vi "UI_Set_ByZone_Stim._Control_State_on_Startup.vi"(8 "Error In":errorcluster, 9 "Regions to mark selected in":u8[](array[numeric]), 10 "All references cluster":T9, 11 "Settings cluster":T1={"Defaults"={"Default User"=0.0, "VISA Resource Name "=""}, "Recording and saving"={"Researcher name"="", "Name prefix"="", "Data post-processing"={"Filter type"=enum."Savitzky-Golay", "Length"=31, "Order"=3}, "Stop at"=0.0, "\"Stop at\" enabled"=FALSE, "Default save folder path"=path "", "Acquisition FPS"=enum."Max"}, "Geometry"={"Cage diameter, mm"=0, "Starting angle MIDFIELD"=0, "Starting angle BORDER"=0, "Radius, mm CENTER"=0, "Radius, mm MIDFIELD"=0, "N segments MIDFIELD"=0, "N segments BORDER"=0, "R-gap, mm"=0.0, "Bridge swap"=FALSE, "Bridge H. offset"=0.0, "Bridge V. offset"=0.0, "Twisted neck"=FALSE, "Alt. magn. orientation"=FALSE}, "IO parameters"={"IO general config."=0, "IO 1 configuration"=0, "IO 2 configuration"=0, "IO 3 configuration"=0, "IO 4 configuration"=0, "Activate ext. RS-232"=0, "IO inversion config."=0, "Sync capability"=1}, "Stimulus presets array"=[{"Event type"=0, "Dur., s"=0.0, "Stim., s"=0.0, "TTL out N"=1, "Set/Clear"=FALSE, "Stim. has been set"=FALSE}, {"Event type"=0, "Dur., s"=0.0, "Stim., s"=0.0, "TTL out N"=1, "Set/Clear"=FALSE, "Stim. has been set"=FALSE}, {"Event type"=0, "Dur., s"=0.0, "Stim., s"=0.0, "TTL out N"=1, "Set/Clear"=FALSE, "Stim. has been set"=FALSE}, {"Event type"=0, "Dur., s"=0.0, "Stim., s"=0.0, "TTL out N"=1, "Set/Clear"=FALSE, "Stim. has been set"=FALSE}, {"Event type"=0, "Dur., s"=0.0, "Stim., s"=0.0, "TTL out N"=1, "Set/Clear"=FALSE, "Stim. has been set"=FALSE}, {"Event type"=0, "Dur., s"=0.0, "Stim., s"=0.0, "TTL out N"=1, "Set/Clear"=FALSE, "Stim. has been set"=FALSE}, {"Event type"=0, "Dur., s"=0.0, "Stim., s"=0.0, "TTL out N"=1, "Set/Clear"=FALSE, "Stim. has been set"=FALSE}, {"Event type"=0, "Dur., s"=0.0, "Stim., s"=0.0, "TTL out N"=1, "Set/Clear"=FALSE, "Stim. has been set"=FALSE}, {"Event type"=0, "Dur., s"=0.0, "Stim., s"=0.0, "TTL out N"=1, "Set/Clear"=FALSE, "Stim. has been set"=FALSE}, {"Event type"=0, "Dur., s"=0.0, "Stim., s"=0.0, "TTL out N"=1, "Set/Clear"=FALSE, "Stim. has been set"=FALSE}, {"Event type"=0, "Dur., s"=0.0, "Stim., s"=0.0, "TTL out N"=1, "Set/Clear"=FALSE, "Stim. has been set"=FALSE}, {"Event type"=0, "Dur., s"=0.0, "Stim., s"=0.0, "TTL out N"=1, "Set/Clear"=FALSE, "Stim. has been set"=FALSE}, {"Event type"=0, "Dur., s"=0.0, "Stim., s"=0.0, "TTL out N"=1, "Set/Clear"=FALSE, "Stim. has been set"=FALSE}, {"Event type"=0, "Dur., s"=0.0, "Stim., s"=0.0, "TTL out N"=1, "Set/Clear"=FALSE, "Stim. has been set"=FALSE}], "Calibration parameters"={"Timing calibration sw/hw"=1.0, "True FPS"=80.0, "Disp. calibration info"=[]}, "Settings loaded OK"=FALSE} {"Calibration parameters"."Disp. calibration info"."Speed, µl per ms" format="%.3g"; "Calibration parameters"."True FPS" format="%.10g"; "Calibration parameters"."Timing calibration sw/hw" format="%.10g"; "Stimulus presets array"."Event type" items=["Stay for N seconds"]; "Stimulus presets array"."TTL out N" items=["1"=1, "2"=2, "1+2"=3]; "Recording and saving"."Data post-processing"."Order" min=3 max=11 step=2; "Recording and saving"."Data post-processing"."Length" min=5 max=301 step=2; "Geometry"."Cage diameter, mm" scale=0.0..340.0}) -> (0 "Error Out":errorcluster, 1 "Regions to mark selected out":u8[](array[numeric]), 2 "All references cluster out":T9, 3 "Regions set for tracking":u8[](array[numeric]), 5 "Settings cluster out":T1={"Defaults"={"Default User"=0.0, "VISA Resource Name "=""}, "Recording and saving"={"Researcher name"="", "Name prefix"="", "Data post-processing"={"Filter type"=enum."Savitzky-Golay", "Length"=31, "Order"=3}, "Stop at"=0.0, "\"Stop at\" enabled"=FALSE, "Default save folder path"=path "", "Acquisition FPS"=enum."Max"}, "Geometry"={"Cage diameter, mm"=0, "Starting angle MIDFIELD"=0, "Starting angle BORDER"=0, "Radius, mm CENTER"=0, "Radius, mm MIDFIELD"=0, "N segments MIDFIELD"=0, "N segments BORDER"=0, "R-gap, mm"=0.0, "Bridge swap"=FALSE, "Bridge H. offset"=0.0, "Bridge V. offset"=0.0, "Twisted neck"=FALSE, "Alt. magn. orientation"=FALSE}, "IO parameters"={"IO general config."=0, "IO 1 configuration"=0, "IO 2 configuration"=0, "IO 3 configuration"=0, "IO 4 configuration"=0, "Activate ext. RS-232"=0, "IO inversion config."=0, "Sync capability"=1}, "Stimulus presets array"=[{"Event type"=0, "Dur., s"=0.0, "Stim., s"=0.0, "TTL out N"=1, "Set/Clear"=FALSE, "Stim. has been set"=FALSE}, {"Event type"=0, "Dur., s"=0.0, "Stim., s"=0.0, "TTL out N"=1, "Set/Clear"=FALSE, "Stim. has been set"=FALSE}, {"Event type"=0, "Dur., s"=0.0, "Stim., s"=0.0, "TTL out N"=1, "Set/Clear"=FALSE, "Stim. has been set"=FALSE}, {"Event type"=0, "Dur., s"=0.0, "Stim., s"=0.0, "TTL out N"=1, "Set/Clear"=FALSE, "Stim. has been set"=FALSE}, {"Event type"=0, "Dur., s"=0.0, "Stim., s"=0.0, "TTL out N"=1, "Set/Clear"=FALSE, "Stim. has been set"=FALSE}, {"Event type"=0, "Dur., s"=0.0, "Stim., s"=0.0, "TTL out N"=1, "Set/Clear"=FALSE, "Stim. has been set"=FALSE}, {"Event type"=0, "Dur., s"=0.0, "Stim., s"=0.0, "TTL out N"=1, "Set/Clear"=FALSE, "Stim. has been set"=FALSE}, {"Event type"=0, "Dur., s"=0.0, "Stim., s"=0.0, "TTL out N"=1, "Set/Clear"=FALSE, "Stim. has been set"=FALSE}, {"Event type"=0, "Dur., s"=0.0, "Stim., s"=0.0, "TTL out N"=1, "Set/Clear"=FALSE, "Stim. has been set"=FALSE}, {"Event type"=0, "Dur., s"=0.0, "Stim., s"=0.0, "TTL out N"=1, "Set/Clear"=FALSE, "Stim. has been set"=FALSE}, {"Event type"=0, "Dur., s"=0.0, "Stim., s"=0.0, "TTL out N"=1, "Set/Clear"=FALSE, "Stim. has been set"=FALSE}, {"Event type"=0, "Dur., s"=0.0, "Stim., s"=0.0, "TTL out N"=1, "Set/Clear"=FALSE, "Stim. has been set"=FALSE}, {"Event type"=0, "Dur., s"=0.0, "Stim., s"=0.0, "TTL out N"=1, "Set/Clear"=FALSE, "Stim. has been set"=FALSE}, {"Event type"=0, "Dur., s"=0.0, "Stim., s"=0.0, "TTL out N"=1, "Set/Clear"=FALSE, "Stim. has been set"=FALSE}], "Calibration parameters"={"Timing calibration sw/hw"=1.0, "True FPS"=80.0, "Disp. calibration info"=[]}, "Settings loaded OK"=FALSE} {"Calibration parameters"."Disp. calibration info"."Speed, µl per ms" format="%.3g"; "Calibration parameters"."True FPS" format="%.10g"; "Calibration parameters"."Timing calibration sw/hw" format="%.10g"; "Stimulus presets array"."Event type" items=["Stay for N seconds"]; "Stimulus presets array"."TTL out N" items=["1"=1, "2"=2, "1+2"=3]; "Recording and saving"."Data post-processing"."Order" min=3 max=11 step=2; "Recording and saving"."Data post-processing"."Length" min=5 max=301 step=2; "Geometry"."Cage diameter, mm" scale=0.0..340.0})   [LabVIEW 2018, in "Tracker.lvlib"]
uses:
  Tracker.lvlib
  Controls/CTL_Settings_cluster.ctl
  Controls/CTL_Filter_selector.ctl
  Controls/CTL_Acquisition_speed_selector.ctl
  Controls/CTL_Segmented_plot_parameters.ctl
  Controls/CTL_IO_params_cluster.ctl
  Controls/CTL_Single_stimulus_setting.ctl
  Controls/CTL_Calibration_parameters.ctl
  Controls/CTL_Dispenser_calibration_info.ctl
  Controls/CTL_All_References.ctl
  Controls/CTL_Controls_References.ctl
  Controls/CTL_Indicators_References.ctl
  Controls/CTL_Panes_and_VIs_References.ctl
  Controls/CTL_Zones_control_and_indicator.ctl
panel:
  in  "Colors for Stim. setup":T13(array[cluster])=[{"Not Selected"=1143775, "Not Selected"=1143775}, {"Not Selected"=14517504, "Not Selected"=14517504}, {"Not Selected"=1976113, "Not Selected"=1976113}, {"Not Selected"=2575993, "Not Selected"=2575993}]
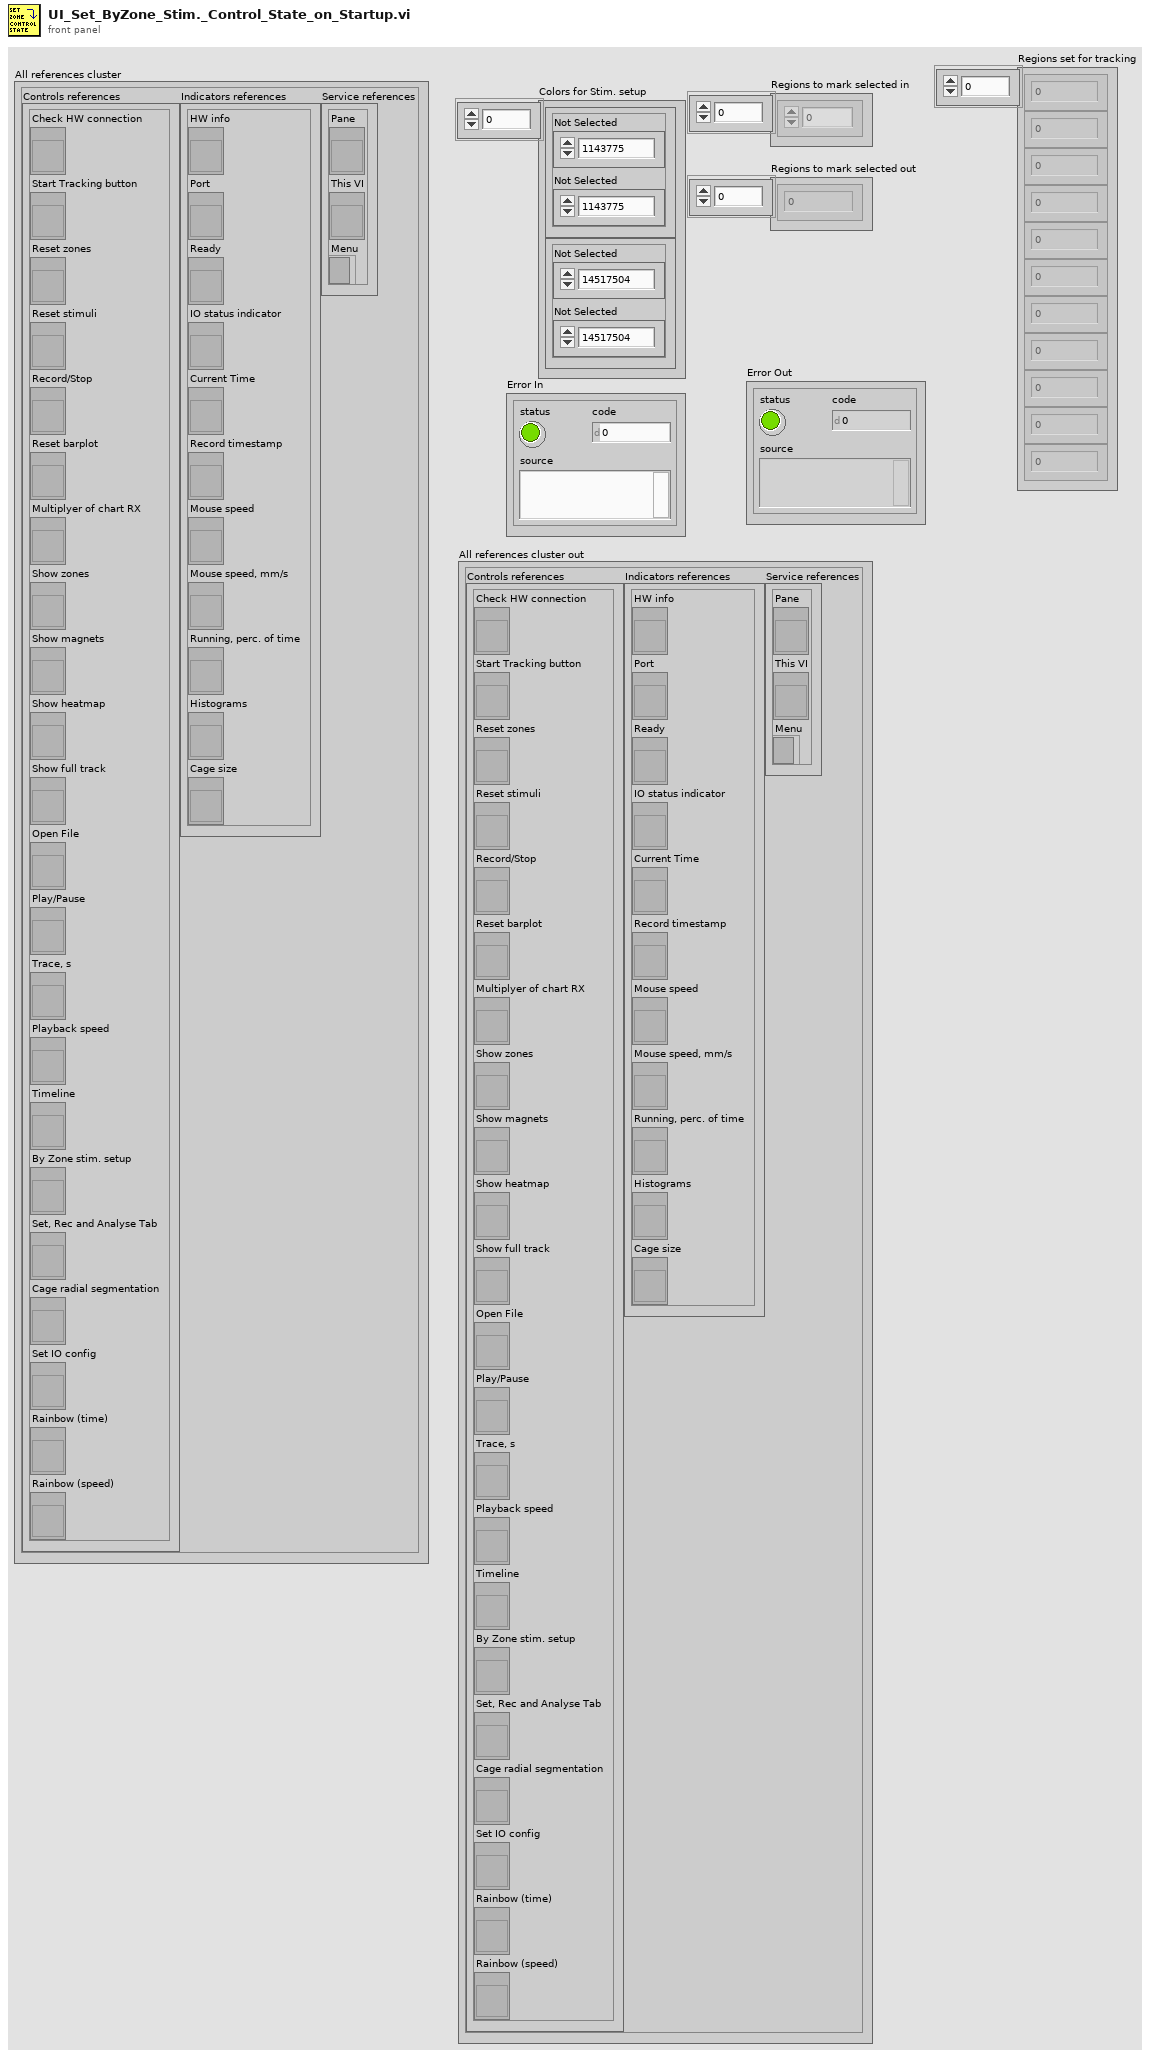
[diagram p1: front panel]
types:
  T1 = typedef "Tracker.lvlib/CTL_Settings_cluster.ctl" = cluster{"Defaults":cluster{"Default User":dbl, "VISA Resource Name ":string}, "Recording and saving":cluster{"Researcher name":string, "Name prefix":string, "Data post-processing":T2, "Stop at":dbl, "\"Stop at\" enabled":bool, "Default save folder path":path, "Acquisition FPS":T3}, "Geometry":T4, "IO parameters":T5, "Stimulus presets array":T6[], "Calibration parameters":T7, "Settings loaded OK":bool}
  T2 = typedef "Tracker.lvlib/CTL_Filter_selector.ctl" = cluster{"Filter type":enum16{"None", "Savitzky-Golay"}, "Length":i32, "Order":i32}
  T3 = typedef "Tracker.lvlib/CTL_Acquisition_speed_selector.ctl" = enum16{"Max", "Optimal", "Eco"}
  T4 = typedef "Tracker.lvlib/CTL_Segmented_plot_parameters.ctl" = cluster{"Cage diameter, mm":u16, "Starting angle MIDFIELD":i16, "Starting angle BORDER":i16, "Radius, mm CENTER":u16, "Radius, mm MIDFIELD":u16, "N segments MIDFIELD":u8, "N segments BORDER":u8, "R-gap, mm":sgl, "Bridge swap":bool, "Bridge H. offset":sgl, "Bridge V. offset":sgl, "Twisted neck":bool, "Alt. magn. orientation":bool}
  T5 = typedef "Tracker.lvlib/CTL_IO_params_cluster.ctl" = cluster{"IO general config.":u16, "IO 1 configuration":u16, "IO 2 configuration":u16, "IO 3 configuration":u16, "IO 4 configuration":u16, "Activate ext. RS-232":u16, "IO inversion config.":u16, "Sync capability":u8}
  T6 = typedef "Tracker.lvlib/CTL_Single_stimulus_setting.ctl" = cluster{"Event type":u16, "Dur., s":sgl, "Stim., s":sgl, "TTL out N":u16, "Set/Clear":bool, "Stim. has been set":bool}
  T7 = typedef "Tracker.lvlib/CTL_Calibration_parameters.ctl" = cluster{"Timing calibration sw/hw":dbl, "True FPS":dbl, "Disp. calibration info":T8}
  T8 = typedef "Tracker.lvlib/CTL_Dispenser_calibration_info.ctl" = cluster{"Channel":u8, "Speed, µl per ms":dbl}[]
  T9 = typedef "Tracker.lvlib/CTL_All_References.ctl" = cluster{"Controls references":T10, "Indicators references":T11, "Service references":T12}
  T10 = typedef "Tracker.lvlib/CTL_Controls_References.ctl" = cluster{"Check HW connection":refnum<vi>, "Start Tracking button":refnum<vi>, "Reset zones":refnum<vi>, "Reset stimuli":refnum<vi>, "Record/Stop":refnum<vi>, "Reset barplot":refnum<vi>, "Multiplyer of chart RX":refnum<vi>, "Show zones":refnum<vi>, "Show magnets":refnum<vi>, "Show heatmap":refnum<vi>, "Show full track":refnum<vi>, "Open File":refnum<vi>, "Play/Pause":refnum<vi>, "Trace, s":refnum<vi>, "Playback speed":refnum<vi>, "Timeline":refnum<vi>, "By Zone stim. setup":refnum<vi>, "Set, Rec and Analyse Tab":refnum<vi>, "Cage radial segmentation":refnum<vi>, "Set IO config":refnum<vi>, "Rainbow (time)":refnum<vi>, "Rainbow (speed)":refnum<vi>}
  T11 = typedef "Tracker.lvlib/CTL_Indicators_References.ctl" = cluster{"HW info":refnum<vi>, "Port":refnum<vi>, "Ready":refnum<vi>, "IO status indicator":refnum<vi>, "Current Time":refnum<vi>, "Record timestamp":refnum<vi>, "Mouse speed":refnum<vi>, "Mouse speed, mm/s":refnum<vi>, "Running, perc. of time":refnum<vi>, "Histograms":refnum<vi>, "Cage size":refnum<vi>}
  T12 = typedef "Tracker.lvlib/CTL_Panes_and_VIs_References.ctl" = cluster{"Pane":refnum<vi>, "This VI":refnum<vi>, "Menu":refnum<k9>}
  T13 = cluster{"Not Selected":u32, "Not Selected":u32}[]
  T14 = typedef "Tracker.lvlib/CTL_Zones_control_and_indicator.ctl" = enum32{"No Selection", "Zone 01", "Zone 02", "Zone 03", "Zone 04", "Zone 05", "Zone 06", "Zone 07", "Zone 08", "Zone 09", "Zone 10", "Zone 11", "Zone 12", "Zone 13"}
  T15 = enum8{"Enabled", "Disabled", "Disabled and Grayed Out"}
  T16 = cluster{"Numeric Control":u32, "Numeric Control":u32}[]
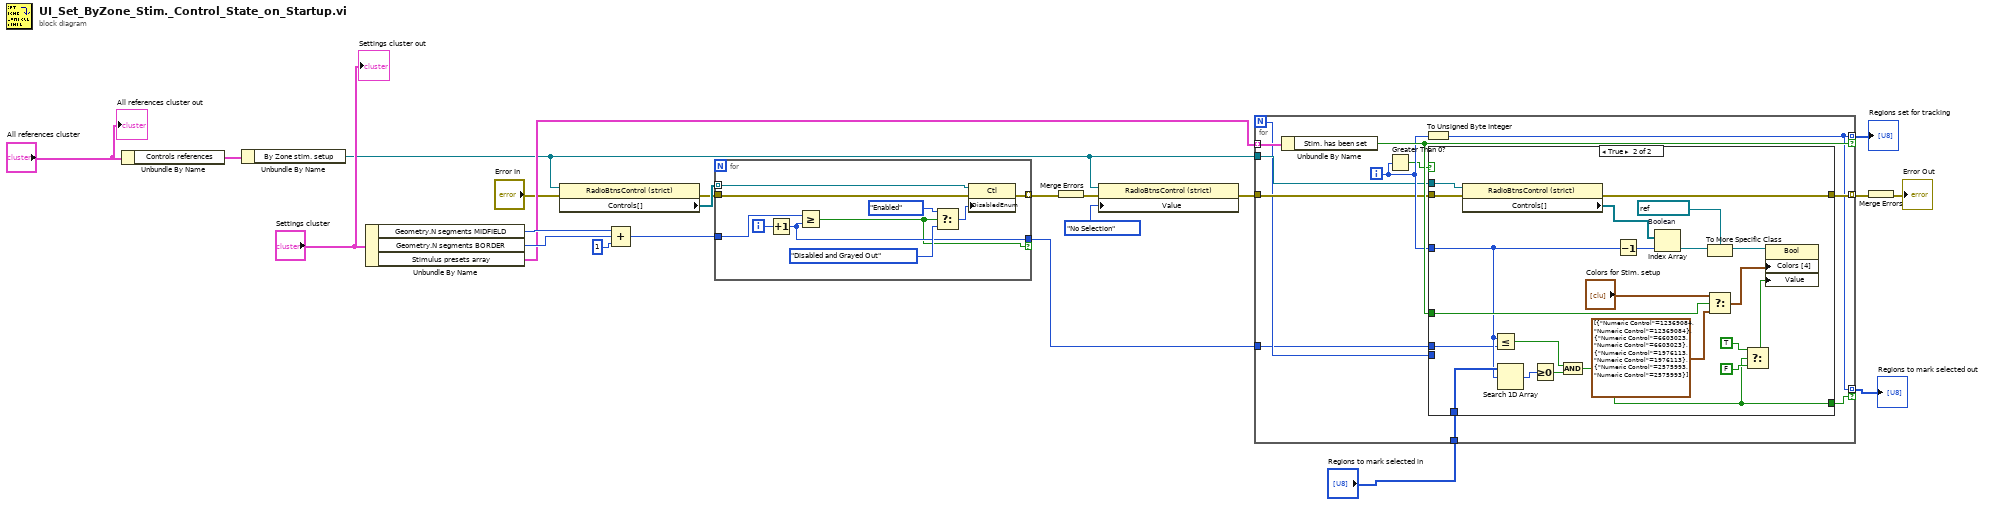
[diagram p0: block diagram]
diagram:
  n1 = Unbundle By Name("All references cluster") -> ("Controls references"=w8:T10)
  n2 = Unbundle By Name(w8) -> ("By Zone stim. setup"=w10:refnum<vi>)
  n3 = Unbundle By Name("Settings cluster") -> ("Geometry.N segments MIDFIELD"=w18:u8, "Geometry.N segments BORDER"=w17:u8, "Stimulus presets array"=w14:T6[])
  n4 = property on="Property Node" class="RadioBtnsControl (strict)"(reference=w10, error in="Error In") -> (error out=w6:errorcluster, "Controls[]"=w22:refnum<vi>[])  [unwired: 1 out]
  n5 = Compound Arithmetic op=ADD(w18, w17, u8 1 ("value")) -> (w15:u8)
  n6 = for {
    tunnel: w22 -> [w32] mode=indexing
    tunnel: w15 -> [w28]
    tunnel: w6 -> [w25]
    tunnel: [w27] -> w20 mode=indexing
    tunnel: [w24] -> w2 if=w23
    i -> [w26]
    n7 = Increment(x=w26) -> (x+1=w24:i32)
    n8 = Greater Or Equal?(x=w28, y=w24) -> (x >= y?=w23:bool)
    n9 = Select(t=T15."Enabled" ("Disabled"), s=w23, f=T15."Disabled and Grayed Out") -> (s? t:f=w30:T15)
    n10 = property class="Ctl"(reference=w32, error in=w25, "DisabledEnum"=w30) -> (error out=w27:errorcluster)  [unwired: 1 out]
  }
  n11 = Merge Errors(w20) -> (w5:errorcluster)
  n12 = property on="Property Node" class="RadioBtnsControl (strict)"(reference=w10, error in=w5, "Value"=CTL_Zones_control_and_indicator."No Selection" ("By Zone stim. setup")) -> (error out=w12:errorcluster)  [unwired: 1 out]
  n13 = for {
    N -> [w36]
    tunnel: w14 -> [w44] mode=indexing
    tunnel: [w34] -> w13 mode=indexing if=w43
    tunnel: w10 -> [w40]
    tunnel: w12 -> [w39]
    tunnel: [w38] -> w11 mode=indexing
    tunnel: "Regions to mark selected in" -> [w37]
    tunnel: w2 -> [w35]
    tunnel: [w34] -> w1 mode=indexing if=w33
    i -> [w42]
    n14 = Unbundle By Name(w44) -> ("Stim. has been set"=w43:bool)
    n15 = Greater Than 0?(x=w42) -> (x > 0?=w41:bool)
    n16 = To Unsigned Byte Integer(number=w42) -> (unsigned 8bit integer=w34:u8)
    n17 = case shown="True" w41 {
      tunnel: w43 -> [_ w67]
      tunnel: w42 -> [_ w48]
      tunnel: w40 -> [_ w60]
      tunnel: w39 -> [w45 w58]
      tunnel: [w45 w57] -> w38
      tunnel: w37 -> [_ w51]
      tunnel: w36 -> [_ _]
      tunnel: w35 -> [_ w47]
      tunnel: [_ w46] -> w33
      frame False {
      }
      frame True {
        w63 = refnum<vi> refnum  # Boolean
        n18 = property on="Property Node" class="RadioBtnsControl (strict)"(reference=w60, error in=w58) -> (error out=w57:errorcluster, "Controls[]"=w65:refnum<vi>[])  [unwired: 1 out]
        n19 = Less Or Equal?(x=w48, y=w47) -> (x <= y?=w49:bool)
        n20 = Search 1D Array(1D array=w51, element=w48) -> (index of element=w50:i32)  [unwired: 1 in]
        n21 = Greater Or Equal To 0?(x=w50) -> (x >= 0?=w52:bool)
        n22 = And(x=w49, y=w52) -> (x .and. y?=w46:bool)
        n23 = Decrement(x=w48) -> (x-1=w56:i32)
        n24 = Index Array(array=w65, index=w56) -> (element=w64:refnum<vi>)
        n25 = To More Specific Class(target class=w63, reference=w64) -> (specific class reference=w62:refnum<vi>)  [unwired: 1 in, 1 out]
        n26 = Select(t="Colors for Stim. setup", s=w67, f=T16 [{"Numeric Control"=12369084, "Numeric Control"=12369084}, {"Numeric Control"=6603023, "Numeric Control"=6603023}, {"Numeric Control"=1976113, "Numeric Control"=1976113}, {"Numeric Control"=2575993, "Numeric Control"=2575993}] ("Colors [4] 2")) -> (s? t:f=w61:T16)
        n27 = Select(t=TRUE, s=w46, f=FALSE) -> (s? t:f=w55:bool)
        n28 = property class="Bool"(reference=w62, "Colors [4]"=w61, "Value"=w55) -> ()  [unwired: 1 in, 2 out]
      }
    }
  }
  "Regions set for tracking" <- w13
  "Regions to mark selected out" <- w1
  n29 = Merge Errors(w11) -> (→"Error Out":errorcluster)
  "All references cluster out" <- "All references cluster"
  "Settings cluster out" <- "Settings cluster"
